vi "Assign GPIO.vi"(8 "error in (no error)":errorcluster, 9 "RX":T1=-1, 10 "TX":T1=-1, 11 "UART in":refnum<class "UART.lvclass">) -> (0 "error out":errorcluster, 3 "UART out":refnum<class "UART.lvclass">)   [LabVIEW 2020, in "CTI.lvlib" / "UART.lvclass"]
uses:
  UART.lvclass
  GPIO Number.ctl
  UART.lvclass/UART.ctl
  CTI.lvlib
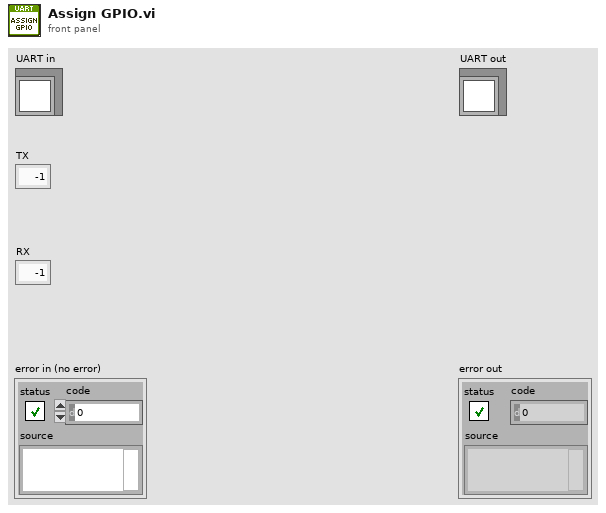
[diagram p1: front panel]
types:
  T1 = typedef "CTI.lvlib/GPIO Number.ctl" = i8
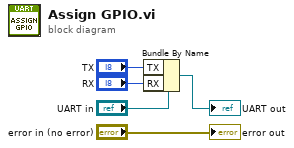
[diagram p0: block diagram]
diagram:
  n1 = Bundle By Name(cluster="UART in", "TX"="TX", "RX"="RX") -> (→"UART out":refnum<class "UART.lvclass">)
  "error out" <- "error in (no error)"
